vi "CALC_CORR_EDEL_WGC.vi"(0 "VISA IN":refnum<visa-resource-name>, 1 "Cutoff Frq.":dbl, 5 "error in":errorcluster, 7 "Channel":i32) -> (14 "VISA Out":refnum<visa-resource-name>, 19 "error out":errorcluster)   [LabVIEW 2018, in "PNA-X.lvlib"]
doc: "CALCulate<cnum>:CORRection:EDELay:WGCutoff <num> \n(Read-Write) Sets the waveguide cutoff frequency used when the electrical delay media is set to \nWAVEguide. (See CALCulate:CORRection:EDELay:MEDium <char>.) \nParameters \n<cnum> Any existing channel number. If unspecified, value is set to 1. \n<num> Waveguide cutoff frequency used with the electrical delay calculation. \nExamples CALC:CORR:EDEL:WGC 18.067 GHz \ncalculate3:correction:edelay:wgcutoff 14.047 ghz \nQuery Syntax CALCulate<cnum>:CORRection:EDELay:WGCutoff? \nReturn Type Numeric \nDefault 45 MHz"
uses:
  PNA-X.lvlib
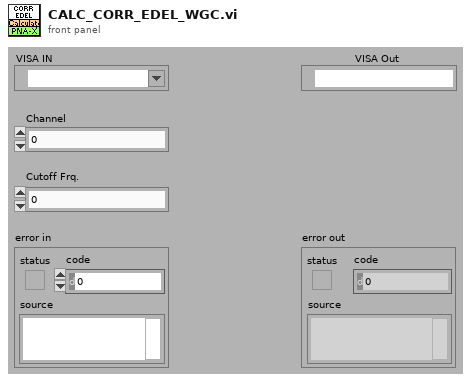
[diagram p1: front panel]
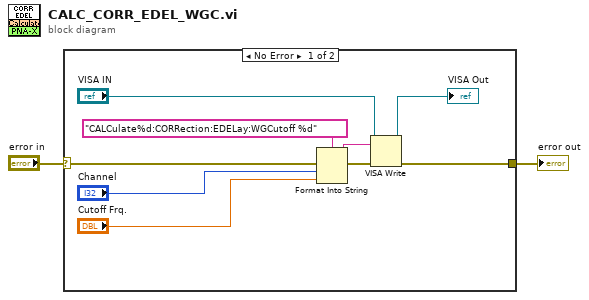
[diagram p0: block diagram]
diagram:
  n1 = case shown="No Error" "error in" {
    selector: "error in" -> [w11 w12]
    tunnel: [w6 w12] -> w1
    frame No Error {
      n2 = Format Into String(format string="CALCulate%d:CORRection:EDELay:WGCutoff %d" ("Cmdline"), error in=w11, "Channel", "Cutoff Frq.") -> (resulting string=w9:string, error out=w10:errorcluster)  [unwired: 1 in]
      n3 = VISA Write(VISA resource name="VISA IN", write buffer=w9, error in (no error)=w10) -> (VISA resource name out=→"VISA Out":refnum<visa-resource-name>, error out=w6:errorcluster)  [unwired: 1 out]
    }
    frame Error {
    }
  }
  "error out" <- w1
